vi "e6.8 (hw7).vi"() -> ()   [LabVIEW 2017]
panel:
  out "Part Available and in Stock?":T1
  in  "Part Looking For and Quantity":cluster{"Part Name":string, "Quantity":dbl}
  # "Chapter 6 (E6.8)"
  # "Enter the part you would like (Hammer, Nails, Wrench, Screwdriver and Screws). If your quantity is lower/equal to the quantity in stock, it will display the information on the right. If they are empty, your quantity is too high."
  # "Putting in Hammer and 100 for Part Name and Quantity respecitvely results in an empty right side."
  # "Patrik Sokolowski"
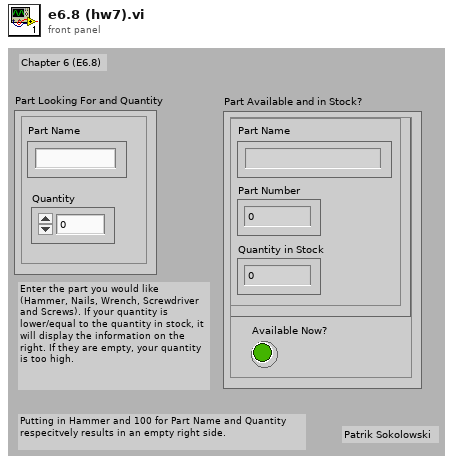
[diagram p1: front panel]
types:
  T1 = cluster{"Cluster":cluster{"Part Name":string, "Part Number":dbl, "Quantity in Stock":dbl}, "Available Now?":bool}
  T2 = cluster{"Part Name":string, "Part Number":dbl, "Quantity":dbl}[]
  T3 = cluster{"Cluster":cluster{"Part Name":string, "Part Number":dbl, "Quantity":dbl}, bool}
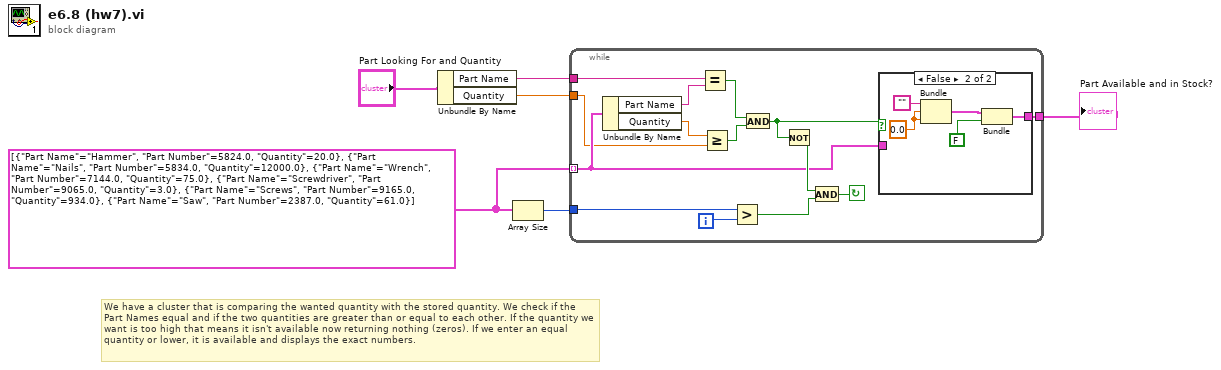
[diagram p0: block diagram]
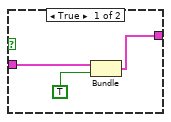
[diagram p2: hidden frame]
diagram:
  w5 = T2 [{"Part Name"="Hammer", "Part Number"=5824.0, "Quantity"=20.0}, {"Part Name"="Nails", "Part Number"=5834.0, "Quantity"=12000.0}, {"Part Name"="Wrench", "Part Number"=7144.0, "Quantity"=75.0}, {"Part Name"="Screwdriver", "Part Number"=9065.0, "Quantity"=3.0}, {"Part Name"="Screws", "Part Number"=9165.0, "Quantity"=934.0}, {"Part Name"="Saw", "Part Number"=2387.0, "Quantity"=61.0}]
  # "We have a cluster that is comparing the wanted quantity with the stored quantity. We check if the Part Names equal and if the two quantities are greater than or equal to each other. If the quantity we want is too high that means it isn't available now returning nothing (zeros). If we enter an equal quantity or lower, it is available and displays the exact numbers."
  n1 = Unbundle By Name("Part Looking For and Quantity") -> ("Part Name"=w1:string, "Quantity"=w2:dbl)
  n2 = Array Size(array=w5) -> (size(s)=w6:i32)
  n3 = while {
    tunnel: w6 -> [w20]
    tunnel: w5 -> [w11] mode=indexing
    tunnel: [w16] -> w3
    tunnel: w2 -> [w7]
    tunnel: w1 -> [w10]
    i -> [w19]
    stop <- w14 continue-if-true
    n4 = Unbundle By Name(w11) -> ("Part Name"=w9:string, "Quantity"=w8:dbl)
    n5 = Equal?(x=w10, y=w9) -> (x = y?=w18:bool)
    n6 = Greater Or Equal?(x=w8, y=w7) -> (x >= y?=w17:bool)
    n7 = Greater?(x=w20, y=w19) -> (0:w12:bool)
    n8 = And(x=w18, y=w17) -> (x .and. y?=w15:bool)
    n9 = Not(x=w15) -> (.not. x?=w13:bool)
    n10 = And(x=w13, y=w12) -> (x .and. y?=w14:bool)
    n11 = case shown="False" w15 {
      tunnel: [w22 w24] -> w16
      tunnel: w11 -> [w21 _]
      frame True {
        n12 = Bundle("Cluster"=w21, TRUE) -> (w22:T3)  [unwired: 1 in]
      }
      frame False {
        w25 = 0.0
        n13 = Bundle("", w25, w25) -> (w27:cluster{string, dbl, dbl})  [unwired: 1 in]
        n14 = Bundle(w27, FALSE) -> (w24:cluster{cluster{string, dbl, dbl}, bool})  [unwired: 1 in]
      }
    }
  }
  "Part Available and in Stock?" <- w3
